vi "draw_boundingbox.vi"(6 "highlight?":bool, 8 "error in (no error)":errorcluster, 9 "depth":dbl[unit], 10 "Image.lvclass":refnum<class "Image.lvclass">, 11 "RoiGeneric in":refnum<class "RoiGeneric.lvclass">) -> (0 "error out":errorcluster, 3 "RoiGeneric out":refnum<class "RoiGeneric.lvclass">)   [LabVIEW 2010, in "RoiGeneric.lvclass"]
uses:
  RoiGeneric.lvclass
  common/classes/Image/Image/Image.lvclass
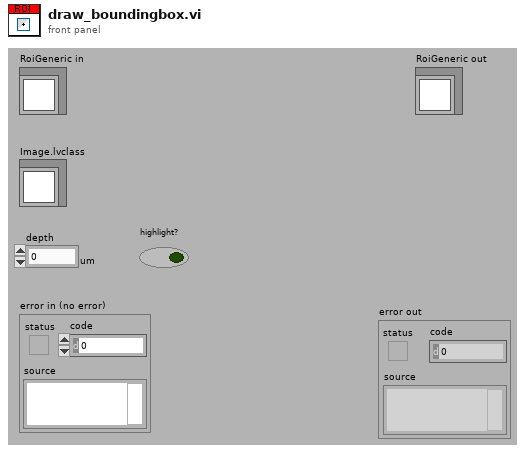
[diagram p1: front panel]
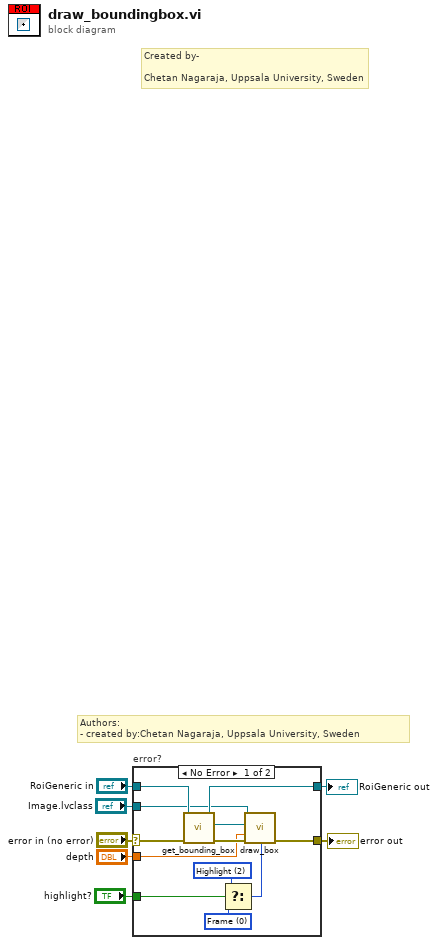
[diagram p0: block diagram]
diagram:
  # "Authors: \n- created by:Chetan Nagaraja, Uppsala University, Sweden"
  # "Created by-\n\nChetan Nagaraja, Uppsala University, Sweden"
  n1 = case "error?" shown="No Error" "error in (no error)" {
    selector: "error in (no error)" -> [w19 w20]
    tunnel: "RoiGeneric in" -> [w18 w21]
    tunnel: "Image.lvclass" -> [w16 _]
    tunnel: "depth" -> [w13 _]
    tunnel: [w14 w20] -> w4
    tunnel: [w17 w21] -> w3
    tunnel: "highlight?" -> [w9 _]
    frame No Error {
      w11 = u32 2 items=["Frame", "Fill", "Highlight"] ("Drawing Mode (Frame)")
      w10 = u32 0 items=["Frame", "Fill", "Highlight"] ("Drawing Mode (Frame)")
      n2 = call-dynamic "get_bounding_box.vi"("error in (no error)"=w19, "RoiGeneric in"=w18) -> ("error out"=w15:errorcluster, "Box.lvclass"=w12:refnum<class "Box.lvclass">, "RoiGeneric out"=w17:refnum<class "RoiGeneric.lvclass">)  [unwired: 7 in]
      n3 = Select(t=w11, s=w9, f=w10) -> (s? t:f=w8:u32)
      n4 = call "draw_box.vi"("Image in"=w16, "Box.lvclass"=w12, "depth"=w13, "error in (no error)"=w15, "drawing mode (Frame)"=w8) -> ("error out"=w14:errorcluster)  [unwired: 9 in, 1 out]
    }
    frame Error {
    }
  }
  "error out" <- w4
  "RoiGeneric out" <- w3
